vi "Version string.vi"(8 "error in":errorcluster) -> (0 "error out":errorcluster, 1 "Development String":string="Development Version ", 2 "IP Address":string="DMILKIE-HP       192.168.0.116", 3 "Version String":string="1.0.0.647              DMILKIE-HP Development Version ")   [LabVIEW 2013]
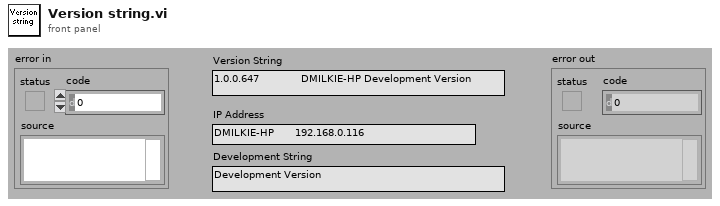
[diagram p1: front panel]
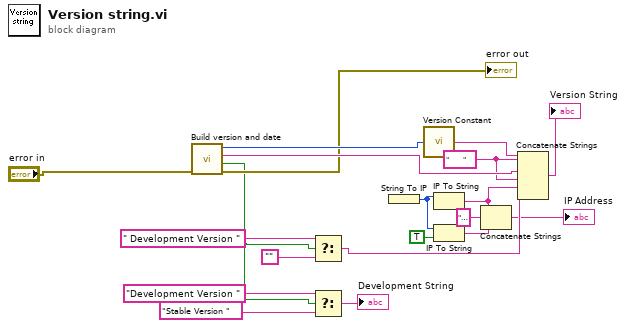
[diagram p0: block diagram]
diagram:
  w15 = "       " ("string")
  n1 = call "Build version and date.vi"("error in"="error in") -> ("error out"=→"error out":errorcluster, "Development?"=w3:bool, "Build date"=w17:string, "Revision"=w13:i32)  [unwired: 7 in]
  n2 = Select(t=" Development Version " ("Default state"), s=w3, f="") -> (s? t:f=w20:string)
  n3 = Select(t="Development Version " ("Default state"), s=w3, f="Stable Version " ("Default state")) -> (s? t:f=→"Development String":string)
  n4 = String To IP() -> (0:w9:u32)  [unwired: 1 in]
  n5 = call "Version Constant.vi"("SCC Revision when built"=w13) -> ("Version"=w12:string)
  n6 = IP To String(2:w9) -> (0:w16:string)  [unwired: 1 in]
  n7 = IP To String(1:TRUE ("dot notation? (F)"), 2:w9) -> (0:w7:string)
  n8 = Concatenate Strings(w16, "       " ("string"), w7) -> (→"IP Address":string)
  n9 = Concatenate Strings(w12, w15, w17, w15, w16, w20) -> (→"Version String":string)
